vi "Calibrate Skew Query.vi"(8 "error in":errorcluster, 11 "Instrument Handle In":i32) -> (0 "error out":errorcluster, 2 "Align Score":i16[](array[numeric]) caption="alignmentScore", 3 "Instrument Handle Out":i32)   [LabVIEW 8.6, in "ZTScopeM.lvlib"]
doc: "Query the instrument's delay code setting for a specific channel. See the instrument calibration manual for more information."
uses:
  ZTScopeM.lvlib
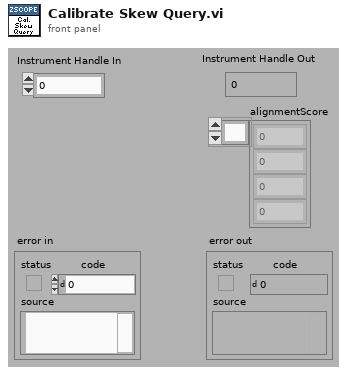
[diagram p1: front panel]
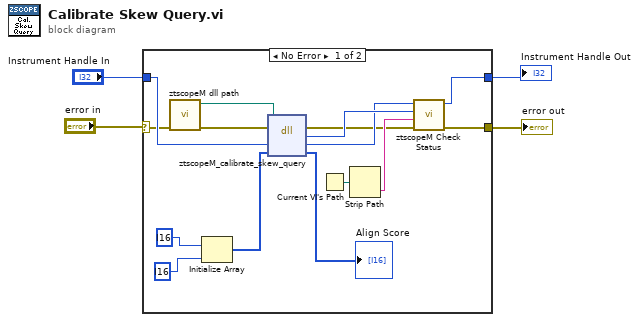
[diagram p0: block diagram]
diagram:
  n1 = case shown="No Error" "error in" {
    selector: "error in" -> [w8 w21]
    tunnel: [w14 w21] -> w1
    tunnel: "Instrument Handle In" -> [w19 w20]
    tunnel: [w13 w20] -> w3
    frame #0 {
      n2 = call "ztscopeM dll path.vi"("error in (no error)"=w8) -> ("error out"=w6:errorcluster, "<instrument>.dll path"=w7:path)  [unwired: 9 in]
      n3 = Initialize Array(i16 ?, i16 ?) -> (w10:i16[])
      n4 = dll-call lib="C:/Program Files (x86)/National Instruments/LabVIEW 2013/instr.lib/ztscopem/ztscopeM.dll" fn="ztscopeM_calibrate_skew_query"(path in=w7, error in=w6, "instrumentHandle"=w19, "alignmentScore"=w10) -> (error out=w5:errorcluster, "return type"=w16:i32, "instrumentHandle"=w15:i32, "alignmentScore"=→"Align Score":i16[])  [unwired: 1 in, 1 out]
      n5 = Current VI's Path() -> (path=w18:path)
      n6 = Strip Path(path=w18) -> (name=w17:string)  [unwired: 1 out]
      n7 = call "ztscopeM Check Status.vi"("error in"=w5, "name of VI"=w17, "status (return code)"=w16, "instrument handle in"=w15) -> ("error out"=w14:errorcluster, "instrument handle out"=w13:i32)  [unwired: 2 in]
    }
    frame #1 {
    }
  }
  "Instrument Handle Out" <- w3
  "error out" <- w1
